vi "timed loop.vi"() -> ()   [LabVIEW 2020]
uses:
  <vilib>/Analysis/Matrix/Datatypes/RealMatrix.ctl
  <vilib>/Platform/TimedLoop/XDataNode/timing_clust.ctl
  <vilib>/Platform/TimedLoop/XDataNode/nitl_modes.ctl
  <vilib>/Platform/TimedLoop/XDataNode/wakeup.ctl
  <vilib>/Analysis/Matrix/Numeric/Conversions/Array To Matrix - RA.vi
  <vilib>/Analysis/Matrix/Numeric/Conversions/Array To Matrix - RA2.vi
  <vilib>/Analysis/Matrix/Numeric/Multiply/Multiply - RM,RM.vi
  <vilib>/platform/TimedLoop/XDataNode/XDataNode.xnode
  <vilib>/Platform/TimedLoop/XDataNode/XDNodeRunTimeDep.lvlib
  <vilib>/Analysis/Matrix/NI_Matrix.lvlib
panel:
  in  "vector size":i32=20
  out "reps":i32
  out "product":T1
  out "average time":dbl
  in  "stop":bool
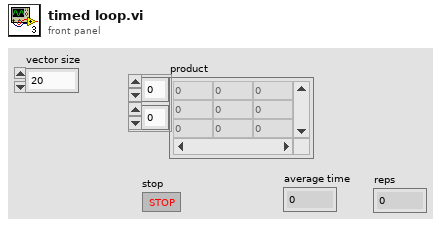
[diagram p1: front panel]
types:
  T1 = typedef "NI_Matrix.lvlib/RealMatrix.ctl" = dbl[][]
  T2 = typedef "XDNodeRunTimeDep.lvlib/timing_clust.ctl" = cluster{"Expected End [f-1]":u64, "Actual End [f-1]":u64, "Finished Late? [f-1]":bool, "Expected End [i-1]":u64, "Actual End [i-1]":u64, "Finished Late? [i-1]":bool, "Expected Start [i]":u64, "Actual Start [i]":u64, "Expected Start [f]":u64, "Actual Start [f]":u64, "Source Name":string, "Structure Name":string, "Period":i64, "Deadline":i64, "Offset":i64, "Start":i64, "Priority":i32, "Timeout":i32, "Mode":T3, "Wakeup Reason":T4, "Error":errorcluster, "Source Type":string, "Secondary Source Type":string, "Global End Time":u64, "Global Start Time":u64, "Frame Duration":u64, "Iteration Duration":u64, "Assigned CPU":i32, "I/O Scan Engine Mode":u32}
  T3 = typedef "XDNodeRunTimeDep.lvlib/nitl_modes.ctl" = enum32{"No Change", "Process missed periods, maintain original phase", "Discard missed periods, maintain original phase", "Process missed periods, ignore original phase", "Discard missed periods, ignore original phase"}
  T4 = typedef "XDNodeRunTimeDep.lvlib/wakeup.ctl" = enum32{"Normal", "Aborted", "Asynchronous wakeup", "Timing source error", "Timed loop error", "Timeout"}
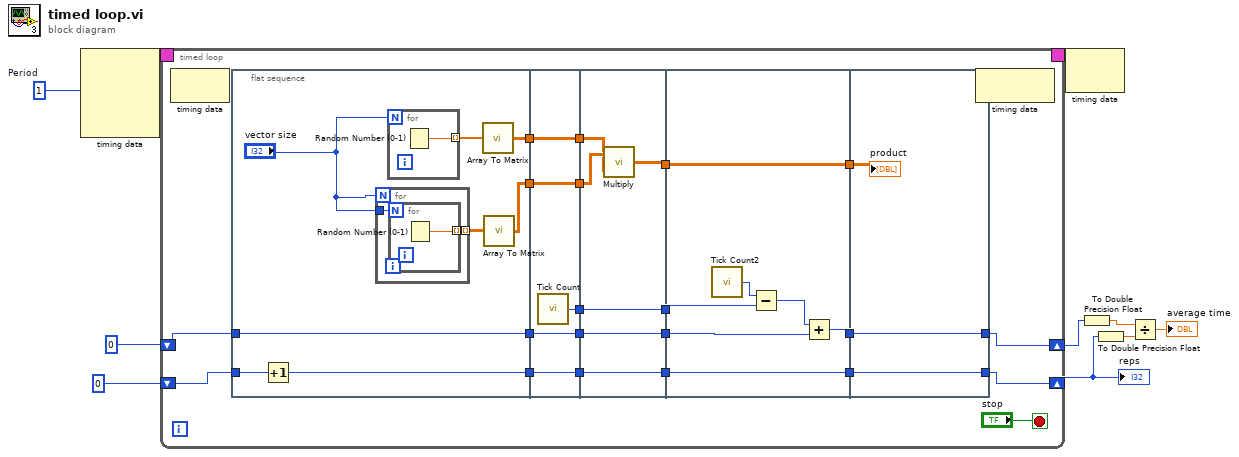
[diagram p0: block diagram]
diagram:
  w6 = i64 1  # Period
  n1 = node-c288(w6) -> (w10:T2)  [unwired: 3 in]
  n2 = timed-loop {
    timing: w10 -> [_]
    timing-out: [_] -> w9
    shift-right: [w29] -> w4
    shift-left: 0 -> [w30]
    shift-right: [w28] -> w2
    shift-left: u32 0 -> [w27]
    stop <- "stop" stop-if-true
    n3 = node-c288() -> ()  [unwired: 1 in, 1 out]
    n4 = flat-sequence {
      tunnel: w30 -> [w39]
      tunnel: [w38] -> w26
      tunnel: [w36] -> w25
      tunnel: w27 -> [w36]
      tunnel: [w35] -> w22
      tunnel: [w33] -> w11
      tunnel: w26 -> [w48]
      tunnel: [w48] -> w24
      tunnel: w25 -> [w47]
      tunnel: [w47] -> w23
      tunnel: w22 -> [w46]
      tunnel: [w46] -> w21
      tunnel: [w45] -> w18
      tunnel: [w44] -> w12
      tunnel: w11 -> [w44]
      tunnel: w24 -> [w54]
      tunnel: [w54] -> w20
      tunnel: w23 -> [w53]
      tunnel: [w53] -> w19
      tunnel: w21 -> [w50]
      tunnel: w18 -> [w52]
      tunnel: [w52] -> w17
      tunnel: [w49] -> w16
      tunnel: w12 -> [w51]
      tunnel: w16 -> [w55]
      tunnel: w17 -> [w58]
      tunnel: w19 -> [w56]
      tunnel: w20 -> [w61]
      tunnel: [w61] -> w15
      tunnel: [w60] -> w14
      tunnel: [w55] -> w13
      tunnel: [w63] -> w28
      tunnel: [w64] -> w29
      tunnel: w15 -> [w64]
      tunnel: w14 -> [w63]
      tunnel: w13 -> [w62]
      frame #0 {
        n5 = Increment(x=w39) -> (x+1=w38:i32)
        n6 = for {
          N: "vector size" -> [_]
          tunnel: [w41] -> w34 mode=indexing
          tunnel: "vector size" -> [w40]
          n7 = for {
            N: w40 -> [_]
            tunnel: [w42] -> w41 mode=indexing
            n8 = Random Number (0-1)() -> (number: 0 to 1=w42:dbl)
          }
        }
        n9 = for {
          N: "vector size" -> [_]
          tunnel: [w43] -> w37 mode=indexing
          n10 = Random Number (0-1)() -> (number: 0 to 1=w43:dbl)
        }
        n11 = call-poly <vilib>:"Array To Matrix.vi"("Real 1D Array"=w37) -> ("Real Matrix (Column Vector)"=w35:T1)
        n12 = call-poly <vilib>:"Array To Matrix.vi"("Real 2D Array"=w34) -> ("Real Matrix"=w33:T1)
      }
      frame #1 {
        n13 = call "Tick Count"() -> ("Tick Count(uSec)"=w45:u32)
      }
      frame #2 {
        n14 = call-poly <vilib>:"Multiply.vi"("Real Matrix B"=w50, "Real Matrix A"=w51) -> ("A * B"=w49:T1)
      }
      frame #3 {
        n15 = call "Tick Count2"() -> ("Tick Count(uSec)"=w59:u32)
        n16 = Subtract(x=w59, y=w58) -> (x-y=w57:u32)
        n17 = Add(x=w57, y=w56) -> (x+y=w60:u32)
      }
      frame #4 {
        "product" <- w62
      }
    }
    n18 = node-c288() -> ()  [unwired: 1 in, 1 out]
  }
  "reps" <- w4
  n19 = node-c288(w9) -> ()  [unwired: 1 out]
  n20 = To Double Precision Float(number=w2) -> (double precision float=w3:dbl)
  n21 = To Double Precision Float(number=w4) -> (double precision float=w5:dbl)
  n22 = Divide(x=w3, y=w5) -> (x/y=→"average time":dbl)
